vi "EEG_2021_099 2D functions of arrays.vi"() -> ()   [LabVIEW 2022 SP3]
panel:
  out "output array":i32[][](array[numeric])
  out "initialized array":i32[][](array[numeric])
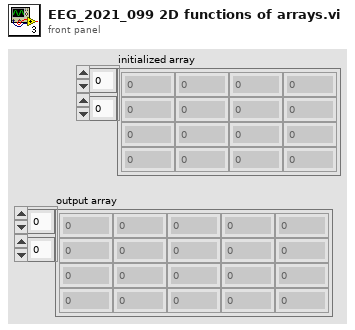
[diagram p1: front panel]
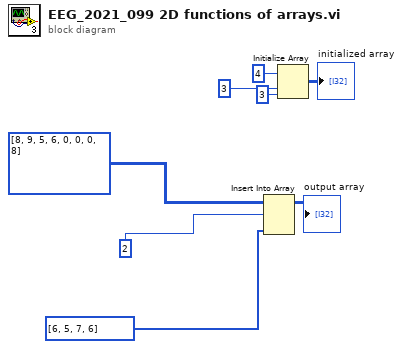
[diagram p0: block diagram]
diagram:
  n1 = Insert Into Array(array=i32[][] [[8, 9, 5, 6], [0, 0, 0, 8]], index (row)=2, new element=i32[] [6, 5, 7, 6]) -> (→"output array":i32[][])  [unwired: 1 in]
  n2 = Initialize Array(4 ("element"), 3 ("dimension size"), 3 ("dimension size")) -> (→"initialized array":i32[][])
